vi "Image Aqq Init.vi"(4 "Error In":errorcluster, 6 "Img In":T1, 7 "Camera":T2) -> (0 "Error Out":errorcluster, 2 "Img Out":T1, 3 "Cam Out":T2)   [LabVIEW 2015]
uses:
  <vilib>/userdefined/High Color/IMAQdx.ctl
  <vilib>/vision/Image Controls.llb/IMAQ Image.ctl
  <vilib>/vision/driver/NI_Vision_Acquisition_Software.lvlib
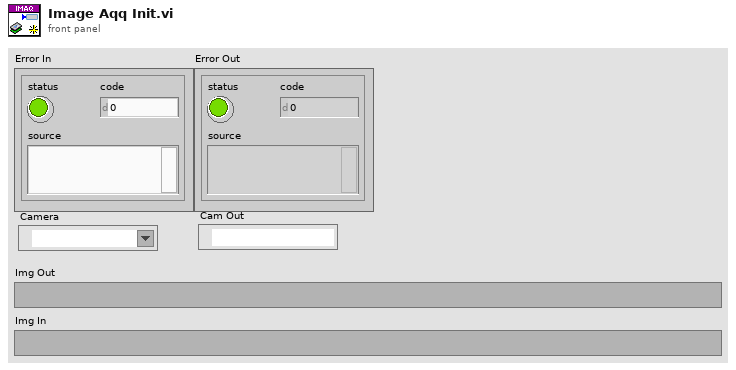
[diagram p1: front panel]
types:
  T1 = typedef "IMAQ Image.ctl" = refnum<image>
  T2 = typedef "IMAQdx.ctl" = refnum<k21>
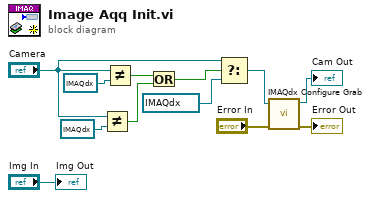
[diagram p0: block diagram]
diagram:
  n1 = Not Equal?(x="Camera", y=T2 " ") -> (x != y?=w1:bool)
  n2 = Not Equal?(x="Camera", y=T2 refnum) -> (x != y?=w2:bool)
  n3 = Or(x=w2, y=w1) -> (x .or. y?=w3:bool)
  n4 = Select(t="Camera", s=w3, f=T2 "cam0") -> (s? t:f=w9:T2)
  n5 = call <vilib>:"IMAQdx Configure Grab.vi"("error in"="Error In", "Session In"=w9) -> ("error out"=→"Error Out":errorcluster, "Session Out"=→"Cam Out":T2)  [unwired: 8 in]
  "Img Out" <- "Img In"
